vi "Report Config Info.vi"(8 "error in (no error)":errorcluster, 11 "Volatus Core in":refnum<class "Volatus Core.lvclass">) -> (0 "error out":errorcluster, 3 "Volatus Core out":refnum<class "Volatus Core.lvclass">)   [LabVIEW 2020, in "Volatus.lvlib" / "Volatus Core.lvclass"]
uses:
  Volatus Core.lvclass
  C:/dev/lv20CE/relink/lv-volatus/Volatus/Module/Module.lvclass
  Volatus Core.lvclass/Volatus Core.ctl
  Module/Module.lvclass/Module.ctl
  Module/Module.lvclass
  VolatusConfig/VolatusConfig/VolatusConfig.lvclass
  C:/dev/lv20CE/relink/lv-volatus/Volatus/Volatus Core/Volatus Core.lvclass
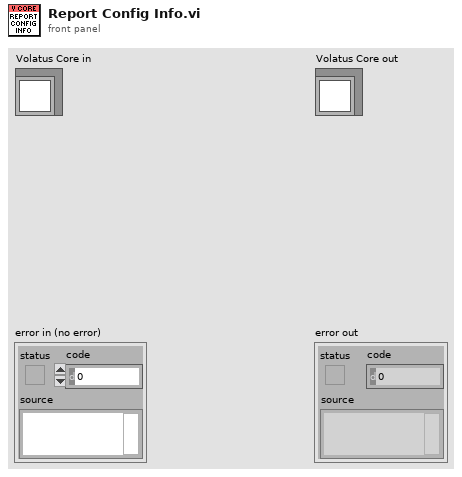
[diagram p1: front panel]
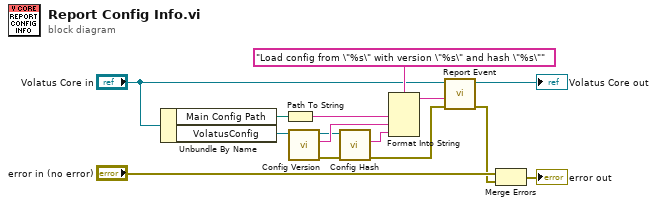
[diagram p0: block diagram]
diagram:
  n1 = Unbundle By Name("Volatus Core in") -> ("Main Config Path"=w8:path, "VolatusConfig"=w14:refnum<class "VolatusConfig.lvclass">)
  n2 = Path To String(path=w8) -> (string=w7:string)
  n3 = call "Config Version.vi"("VolatusConfig in"=w14) -> ("error out"=w3:errorcluster, "Config Version"=w13:string, "VolatusConfig out"=w4:refnum<class "VolatusConfig.lvclass">)  [unwired: 8 in]
  n4 = call "Config Hash.vi"("error in (no error)"=w3, "VolatusConfig in"=w4) -> ("error out"=w1:errorcluster, "Config Hash"=w2:string)  [unwired: 7 in, 1 out]
  n5 = Format Into String(format string="Load config from \"%s\" with version \"%s\" and hash \"%s\"", w7, w13, w2) -> (resulting string=w12:string)  [unwired: 2 in, 1 out]
  n6 = call "Report Event.vi"("error in (no error)"=w1, "Message"=w12, "Module in"="Volatus Core in") -> ("error out"=w5:errorcluster, "Module out"=→"Volatus Core out":refnum<class "Volatus Core.lvclass">)  [unwired: 7 in]
  n7 = Merge Errors("error in (no error)", w5) -> (→"error out":errorcluster)
